vi "OE1022D_USB_Query Data.vi"(0 "VISA resource name":refnum<visa-resource-name>, 11 "Error in (no error)":errorcluster caption="error out（no error）") -> (3 "Buffer Count":u8, 4 "VISA resource  out":refnum<visa-resource-name>, 6 "CH A_Parameter Values":T2, 8 "CH B_Parameter Values":T2, 10 "Total Date Array":dbl[][](array[numeric]), 13 "PLL&Overload":T1, 14 "Output String":string, 15 "Error out":errorcluster caption="error out")   [LabVIEW 2011]
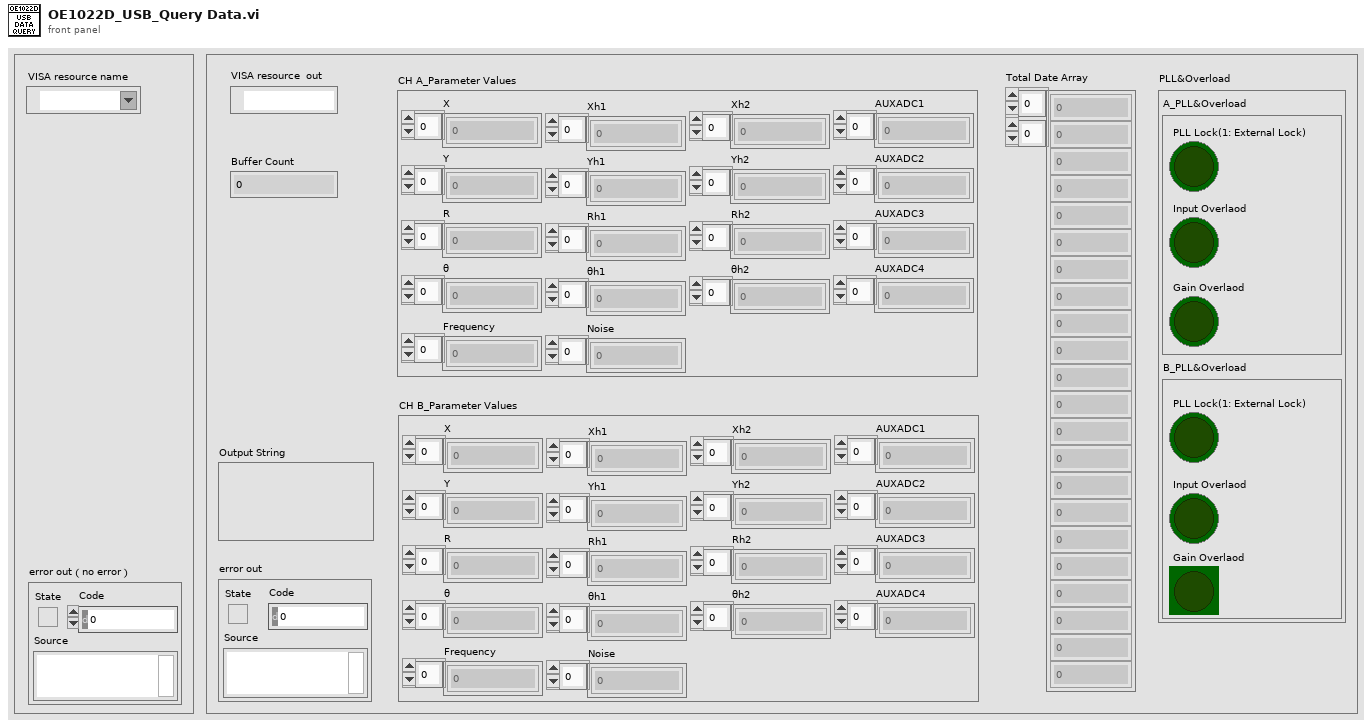
[diagram p1: front panel]
types:
  T1 = cluster{"A_PLL&Overload":cluster{"PLL Lock(1: External Lock)":bool, "Input Overlaod":bool, "Gain Overlaod":bool}, "B_PLL&Overload":cluster{"PLL Lock(1: External Lock)":bool, "Input Overlaod":bool, "Gain Overlaod":bool}}
  T2 = cluster{"X":dbl[], "Y":dbl[], "R":dbl[], "θ":dbl[], "Noise":dbl[], "Frequency":dbl[], "Xh1":dbl[], "Yh1":dbl[], "Rh1":dbl[], "θh1":dbl[], "Xh2":dbl[], "Yh2":dbl[], "Rh2":dbl[], "θh2":dbl[], "AUXADC1":dbl[], "AUXADC2":dbl[], "AUXADC3":dbl[], "AUXADC4":dbl[]}
  T3 = enum16{"ISRC", "IGND", "ICPL", "ILIN", "PHAS", "FMOD", "RSLP", "FREQ", "SWPT", "SLLM", "SULM", "SSLL", "SSLG", "STLM", "SWRM", "IRNG", "SENS", "RMOD", "OFLT", "OFSL", "SYNC", "DMOD", "HARM", "DARB", "SWVT", "SLVL", "SVLL", "SVUL", "SVSL", "SVSG", "SVTM", "SVRM", "RALL", "SNAP", "OUTP", "OAUX", "COUT", "CAUX", "COFP", "CEXP", "FPOP", "OEXP", "*IDN", "*RST", "OVLD", "INOV", "GNOV", "*PLL", "SSET", "RSET", "AGAN", "APHS", "ARSV", "ASCL", "EQCD", "EQCS", "SPED", "SRAT", "SLEN", "SSLE", "STRG", "SPRM", "STRD", "PAUS", "REST", "SPTS", "TRCA", "TEMP", "RSTU", "IHNZ", "DEQU", "SADD", "ARNG", "CSPE", "ISRCD", "IGNDD", "ICPLD", "ILIND", "PHASD", "FMODD", "RSLPD", "FREQD", "SWPTD", "SLLMD", "SULMD", "SSLLD", "SSLGD", "STLMD", "SWRMD", "SENSD", "RMODD", "OFLTD", "OFSLD", "SYNCD", "HARMD", "EQCDD", "EQCSD", "SNAPD", "OUTPD", "SWVTD", "SLVLD", "SVLLD", "SVULD", "SVSLD", "SVSGD", "SVTMD", "SVRMD", "SVDCD", "ARSVD", "AGAND", "APHSD", "ASCLD", "FPOPD", "CAUXD", "OEXPD", "SPEDD", "SRATD", "SLEND", "SSLED", "STRGD", "SPRMD", "STRDD", "PAUSD", "RESTD", "SPTSD", "TRCAD", "*IDND", "*RSTD", "INOVD", "GNOVD", "*PLLD", "SSETD", "RSETD", "RALLD"}
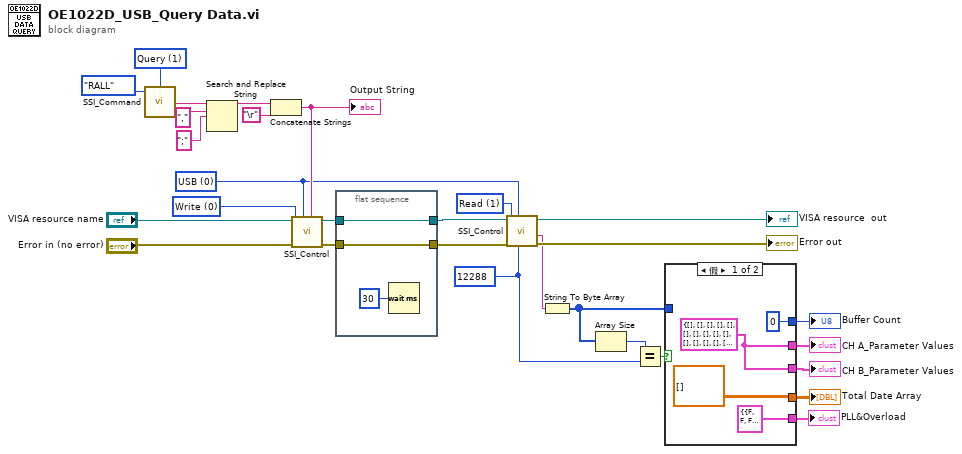
[diagram p0: block diagram]
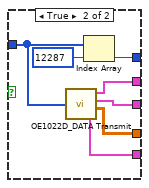
[diagram p2: hidden frame]
diagram:
  w21 = u16 1 items=["Set", "Query"] ("Opera")
  w23 = u16 0 items=["USB", "RS232", "GPIB", "Ethernet"] ("Remote Mode")
  w4 = u32 12288 ("Number of bytes")
  w25 = u16 1 items=["Write", "Read"] ("Control")
  w26 = u16 0 items=["Write", "Read"] ("Control")
  n1 = call "SSI_Command.vi"("Opera"=w21, "Command Type"=T3."RALL") -> ("Output string"=w20:string)  [unwired: 2 in]
  n2 = Search and Replace String(input string=w20, search string="," ("搜索字符串"), replace string=";") -> (result string=w16:string)  [unwired: 5 in, 3 out]
  n3 = Concatenate Strings(w16, "\r") -> (w24:string)
  "Output String" <- w24
  n4 = call "SSI_Control.vi"("Write Buffer"=w24, "Remote Mode"=w23, "Error in (no error)"="Error in (no error)", "Control"=w26, "VISA resource name"="VISA resource name") -> ("Error out"=w7:errorcluster, "VISA resource  out"=w9:refnum<visa-resource-name>)  [unwired: 3 in, 2 out]
  n5 = flat-sequence {
    tunnel: [w32] -> w8
    tunnel: w9 -> [w32]
    tunnel: w7 -> [w31]
    tunnel: [w31] -> w6
    frame #0 {
      n6 = Wait (ms)(milliseconds to wait=u32 30 ("等待时间（毫秒）")) -> ()  [unwired: 1 out]
    }
  }
  n7 = call "SSI_Control.vi"("Number of bytes"=w4, "Remote Mode"=w23, "Error in (no error)"=w6, "Control"=w25, "VISA resource name"=w8) -> ("Error out"=→"Error out":errorcluster, "Read Buffer"=w14:string, "VISA resource  out"=→"VISA resource  out":refnum<visa-resource-name>)  [unwired: 3 in, 1 out]
  n8 = String To Byte Array(string=w14) -> (unsigned byte array=w2:u8[])
  n9 = Array Size(array=w2) -> (size(s)=w3:i32)
  n10 = Equal?(x=w3, y=w4) -> (x = y?=w5:bool)
  n11 = case shown="假" w5 {
    tunnel: w2 -> [_ w41]
    tunnel: [u8 0 w42] -> w13
    tunnel: [w34 w40] -> w12
    tunnel: [w34 w39] -> w11
    tunnel: [dbl[][] [] ("Total Date Array") w38] -> w10
    tunnel: [T1 {"A_PLL&Overload"={"PLL Lock(1: External Lock)"=FALSE, "Input Overlaod"=FALSE, "Gain Overlaod"=FALSE}, "B_PLL&Overload"={"PLL Lock(1: External Lock)"=FALSE, "Input Overlaod"=FALSE, "Gain Overlaod"=FALSE}} ("PLL&Overload") w37] -> w1
    frame False {
      w34 = T2 {"X"=[], "Y"=[], "R"=[], "θ"=[], "Noise"=[], "Frequency"=[], "Xh1"=[], "Yh1"=[], "Rh1"=[], "θh1"=[], "Xh2"=[], "Yh2"=[], "Rh2"=[], "θh2"=[], "AUXADC1"=[], "AUXADC2"=[], "AUXADC3"=[], "AUXADC4"=[]} ("CH A_Parameter Values")
    }
    frame True {
      n12 = call "OE1022D_DATA Transmit.vi"("Input Data"=w41) -> ("CH A_Parameter Values"=w40:T2, "CH B_Parameter Values"=w39:T2, "Total Date Array"=w38:dbl[][], "PLL&Overload"=w37:T1)
      n13 = Index Array(array=w41, index=12287 ("索引")) -> (element=w42:u8)
    }
  }
  "CH A_Parameter Values" <- w12
  "CH B_Parameter Values" <- w11
  "Buffer Count" <- w13
  "Total Date Array" <- w10
  "PLL&Overload" <- w1
